vi "niRFUtil WFM Parse Waveform - Chunk (complex wfm).vi"(3 "Duration (Inf)":dbl=inf format="%^.6e", 4 "Start (-Inf)":dbl=-inf format="%^.6e", 5 "Waveform In":T1 {"y" format="%.2f"; "dx" format="%^.2e"; "x0" format="%^.2e"}) -> (2 "Waveform Out":T1 {"y" format="%.2f"; "dx" format="%^.2e"; "x0" format="%^.2e"})   [LabVIEW 2015, in "niRFUtil.lvlib"]
doc: "(c) Copyright 2006, National Instruments, Inc. This VI may not be duplicated, sold, or distributed without written consent from National Instruments."
uses:
  niRFUtil.lvlib
  Includes/niRFUtil INC Complex Waveform.ctl
  Includes/niRFUtil INC Complex Array.ctl
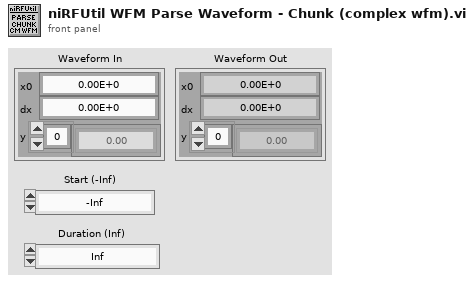
[diagram p1: front panel]
types:
  T1 = typedef "niRFUtil.lvlib/niRFUtil INC Complex Waveform.ctl" = cluster{"x0":dbl, "dx":dbl, "y":T2}
  T2 = typedef "niRFUtil.lvlib/niRFUtil INC Complex Array.ctl" = csg[]
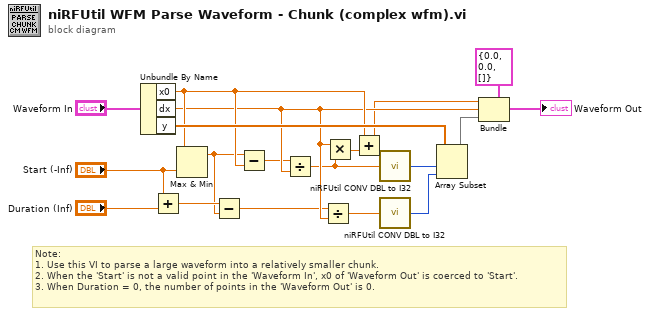
[diagram p0: block diagram]
diagram:
  # "Note:\n1. Use this VI to parse a large waveform into a relatively smaller chunk.\n2. When the 'Start' is not a valid point in the 'Waveform In', x0 of 'Waveform Out' is coerced to 'Start'.\n3. When Duration = 0, the number of points in the 'Waveform Out' is 0."
  n1 = Unbundle By Name("Waveform In") -> ("x0"=w14:dbl, "dx"=w12:dbl, "y"=w15:T2)
  n2 = Add(x="Start (-Inf)", y="Duration (Inf)") -> (x+y=w9:dbl)
  n3 = Max & Min(x=w14, y="Start (-Inf)") -> (max(x,y)=w8:dbl)  [unwired: 1 out]
  n4 = Subtract(x=w9, y=w8) -> (x-y=w7:dbl)
  n5 = Subtract(x=w8, y=w14) -> (x-y=w10:dbl)
  n6 = Divide(x=w10, y=w12) -> (x/y=w6:dbl)
  n7 = Divide(x=w7, y=w12) -> (x/y=w4:dbl)
  n8 = Multiply(x=w12, y=w6) -> (x*y=w16:dbl)
  n9 = Add(x=w14, y=w16) -> (x+y=w11:dbl)
  n10 = call "niRFUtil CONV DBL to I32.vi"("Numeric (DBL)"=w6) -> ("Numeric (I32)"=w5:i32)  [unwired: 14 in]
  n11 = call "niRFUtil CONV DBL to I32.vi"("Numeric (DBL)"=w4) -> ("Numeric (I32)"=w3:i32)  [unwired: 14 in]
  n12 = Array Subset(array=w15, index=w5, length=w3) -> (w13:T2)
  n13 = Bundle(cluster=T1 {"x0"=0.0, "dx"=0.0, "y"=[]} ("Waveform Out 2"), "x0"=w11, "dx"=w12, "y"=w13) -> (→"Waveform Out":T1)
